vi "Close2DGraph.vi"(8 "error in (no error)":errorcluster caption="entrée d'erreur (pas d'erreur)", 10 "GraphIndexArr":i32, 11 "Interface en entrée":refnum<class "Interface.lvclass"> caption="DNL_LabVIEW Object in") -> (0 "error out":errorcluster caption="sortie d'erreur", 3 "Interface en sortie":refnum<class "Interface.lvclass"> caption="DNL_LabVIEW Object out")   [LabVIEW 2019, in "Interface.lvclass"]
uses:
  Interface.lvclass
  Interface.lvclass/Interface.ctl
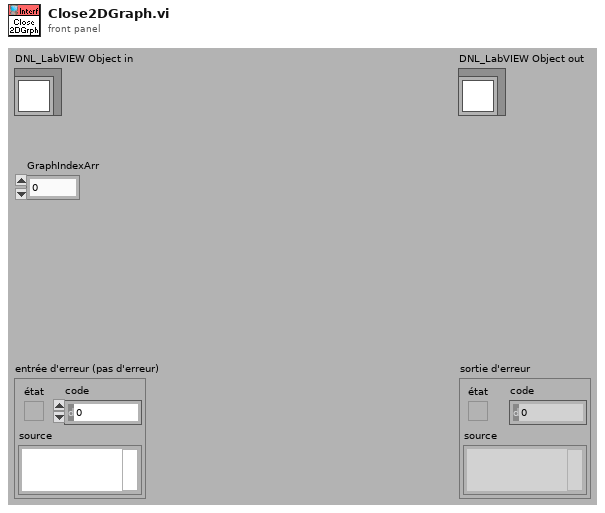
[diagram p1: front panel]
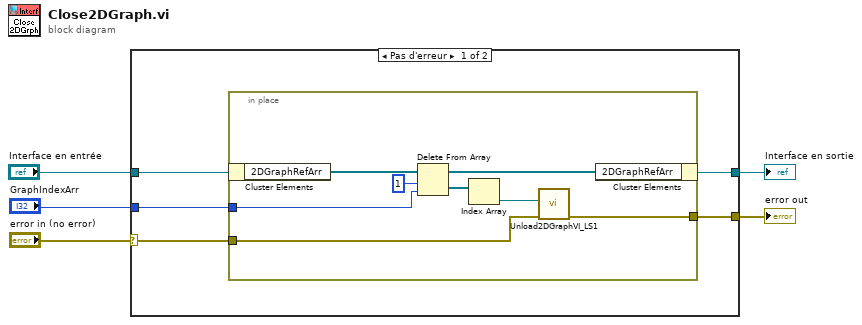
[diagram p0: block diagram]
diagram:
  n1 = case shown="Pas d'erreur" "error in (no error)" {
    selector: "error in (no error)" -> [w8 w20]
    tunnel: [w6 w20] -> w4
    tunnel: [w7 w19] -> w2
    tunnel: "Interface en entrée" -> [w10 w19]
    tunnel: "GraphIndexArr" -> [w9 _]
    frame No Error {
      n2 = in-place {
        in-place-border: w9 -> [w13]
        in-place-border: w8 -> [w12]
        in-place-border: [w11] -> w6
        n3 = in-place-cluster #1(w10) -> ("2DGraphRefArr"=w18:refnum<vi>[])
        n4 = Delete From Array(array=w18, length=1 ("longueur"), index=w13) -> (deleted portion=w15:refnum<vi>[], array with subset deleted=w17:refnum<vi>[])
        n5 = Index Array(array=w15) -> (element=w14:refnum<vi>)  [unwired: 1 in]
        n6 = call "Unload2DGraphVI_LS1.vi"("ErrorIn(No Error)"=w12, "GraphRef"=w14) -> ("sortie d'erreur"=w11:errorcluster)  [unwired: 9 in]
        n7 = in-place-cluster #1("2DGraphRefArr"=w17) -> (w7:refnum<class "Interface.lvclass">)
      }
    }
    frame Error {
    }
  }
  "error out" <- w4
  "Interface en sortie" <- w2
